vi "random sub.vi"() -> (3 "Numeric":dbl)   [LabVIEW 2014]
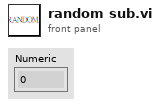
[diagram p1: front panel]
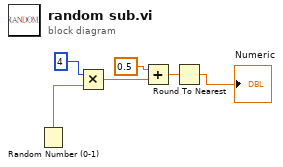
[diagram p0: block diagram]
diagram:
  n1 = Random Number (0-1)() -> (number: 0 to 1=w1:dbl)
  n2 = Multiply(x=i8 4, y=w1) -> (x*y=w3:dbl)
  n3 = Add(x=0.5, y=w3) -> (x+y=w5:dbl)
  n4 = Round To Nearest(number=w5) -> (nearest integer value=→"Numeric":dbl)
